vi "Diagnostics.Cleanup.vi"(8 "error in (no error)":errorcluster, 11 "State Variables":T1={"Comm"=refnum, "Parameters"={"Properties"={"Name"="", "CAN"={"CAN Interface"=enum."CAN1", "Baud Rate"=0, "Diagnostic Protocol"=enum."GMLAN", "Transport Protocol"=enum."ISO TP - Normal Mode", "Transmit ID"=0, "Receive ID"=0, "Transmit Extension"=2, "Receive Extension"=1, "Receive UUDT ID"=0, "Enable Stream"=TRUE, "VW TP Channel ID"=0, "Security"={"Source DLL Path"=path "", "Security Level"=0, "Target DLL Path"=path ""}, "Fill Frame"=FALSE, "Fill Byte"=255, "Termination"=FALSE}, "986x"={"Enable"=FALSE, "RIO Device"=0, "Bitfile"=path ""}, "Reads"=[], "Frames Lookup"=variant(enum16{"GMLAN", "KWP-2000", "UDS"} enum."GMLAN"), "Writes"=[], "DPIDs"=[], "DPID Lookup"=variant(u32 0), "DTC descriptor"={"DTC Byte Length"=2, "Status Byte Length"=1, "Add Data Byte Length"=1, "Byte Order"=enum."Motorola"}, "Created DTCs"=0}}, "ADCS Connection"={"Diag CAN Handle"=0, "Transport Protocol"=enum."ISO TP - Normal Mode", "Receive Address Extension"=0, "Transmit Address Extension"=0, "Receive CAN Id"=0, "Transmit CAN Id"=0, "Diag CAN Queue"=refnum, "Log Frames ?"=FALSE, "My TP Address"=0, "Other TP Address"=0, "T1"=0, "T2"=0, "T3"=0, "T4"=0, "Tx SN"=0, "Block Size"=0, "Rx SN"=0, "VW TP Initialized?"=FALSE, "Tx block no"=0, "baud rate"=0, "Interface"="", "Channel Diag CAN Handle"=0, "UDP Connection ID"=refnum, "TCP Connection ID"=refnum, "Target IP Addr"=0, "Source Address"=0, "Target Address"=0, "Send Header NACK?"=FALSE, "DLL Handle"=0, "NAD"=0, "Time Stamp read first"=0.0, "Time Stamp read last"=0.0, "Time Stamp write first"=0.0, "Time Stamp write last"=0.0, "Time Stamp write"=0.0, "Time Stamp read"=0.0}, "XNET References"={"Database"="", "GMLAN DPID Session"="", "Cluster"=""}, "XNETEngine (GMLAN)"=refnum, "Process"=refnum, "Reads"=refnum, "Writes"=refnum, "Cmds"=refnum, "DTCs"=refnum, "DTC Count"=refnum, "Status"=refnum, "Triggers"=refnum} {"Parameters"."Properties"."Writes"."Signals"."Byte Order" items=["Little Endian", "Big Endian"]; "Parameters"."Properties"."Writes"."Signals"."Data Type" items=["Signed", "Unsigned", "IEEE Float"]; "Parameters"."Properties"."CAN"."Fill Byte" format="%.0x"; "Parameters"."Properties"."CAN"."VW TP Channel ID" format="%.0x"; "Parameters"."Properties"."CAN"."Receive UUDT ID" format="%.0x"; "Parameters"."Properties"."CAN"."Receive Extension" format="%.0x"; "Parameters"."Properties"."CAN"."Transmit Extension" format="%.0x"; "Parameters"."Properties"."CAN"."Receive ID" format="%.0x"; "Parameters"."Properties"."CAN"."Transmit ID" format="%.0x"; "Parameters"."Properties"."Reads"."Signals"."Byte Order" items=["Little Endian", "Big Endian"]; "Parameters"."Properties"."Reads"."Signals"."Data Type" items=["Signed", "Unsigned", "IEEE Float"]}) -> (0 "error out":errorcluster)   [LabVIEW 2015, in "Diagnostics Addon Engine.lvlib"]
uses:
  Diagnostics Addon Engine.lvlib
  Types/Diagnostics.State.ctl
  <vilib>/NI/NIVS Inline Async API/_VS Inline Async API/Process/Process.lvclass
  <vilib>/NI/NIVS Addon Network Comm/Engine/VeriStand Comm.lvclass
  Shared/Types/SysDef.Compile.ctl
  Shared/Types/SysDef.Compile.Properties.ctl
  Shared/Types/CAN.ctl
  Shared/Types/CAN.Interface.ctl
  Shared/Types/Protocol.ctl
  Shared/Types/Transport.ctl
  Shared/Types/Security.ctl
  Shared/Types/986x.ctl
  Shared/Types/Frame.Compile.ctl
  Shared/Types/Type.ctl
  Shared/Types/Signal.ctl
  Shared/Types/DPID.ctl
  Shared/Types/DPID.Rate.ctl
  Shared/Types/DTCDescriptor.ctl
  <vilib>/Automotive Diagnostic Command Set/Diagnostic Transport.llb/Diag Reference.ctl
  <vilib>/Automotive Diagnostic Command Set/Diagnostic Transport.llb/Transport Protocol Selector.ctl
  <vilib>/Automotive Diagnostic Command Set/Diagnostic Transport.llb/Diag CAN Frame Log.ctl
  Types/XNET.Refs.ctl
  <vilib>/NI/AMC/Message Queue.ctl
  <vilib>/NI/AMC/Message.ctl
  <vilib>/NI/Tools/Keyed Array/KeyedArray.ctl
  <vilib>/NI/NIVS Inline Async API/_Data Access Engine/Access Type Classes/Write/Write.lvclass
  <vilib>/NI/NIVS Inline Async API/_Data Access Engine/Access Type Classes/Read/Read.lvclass
  <vilib>/NI/NIVS Inline Async API/_Data Access Engine/Access Type Classes/ReadWrite/ReadWrite.lvclass
  <vilib>/xnet/xnet.llb/XNET Database Close (Database).vi
  <vilib>/xnet/xnet.llb/XNET Database Delete (Cluster).vi
  Shared/SubVIs/Constants.vi
  <vilib>/addons/Automotive Diagnostic Command Set/NI_Automotive Diagnostic Command Set.lvlib
  <vilib>/NI/AMC/AMC.lvlib
  Shared/Diagnostics Addon Shared.lvlib
  <vilib>/NI/Tools/Keyed Array/Tools_KeyedArray.lvlib
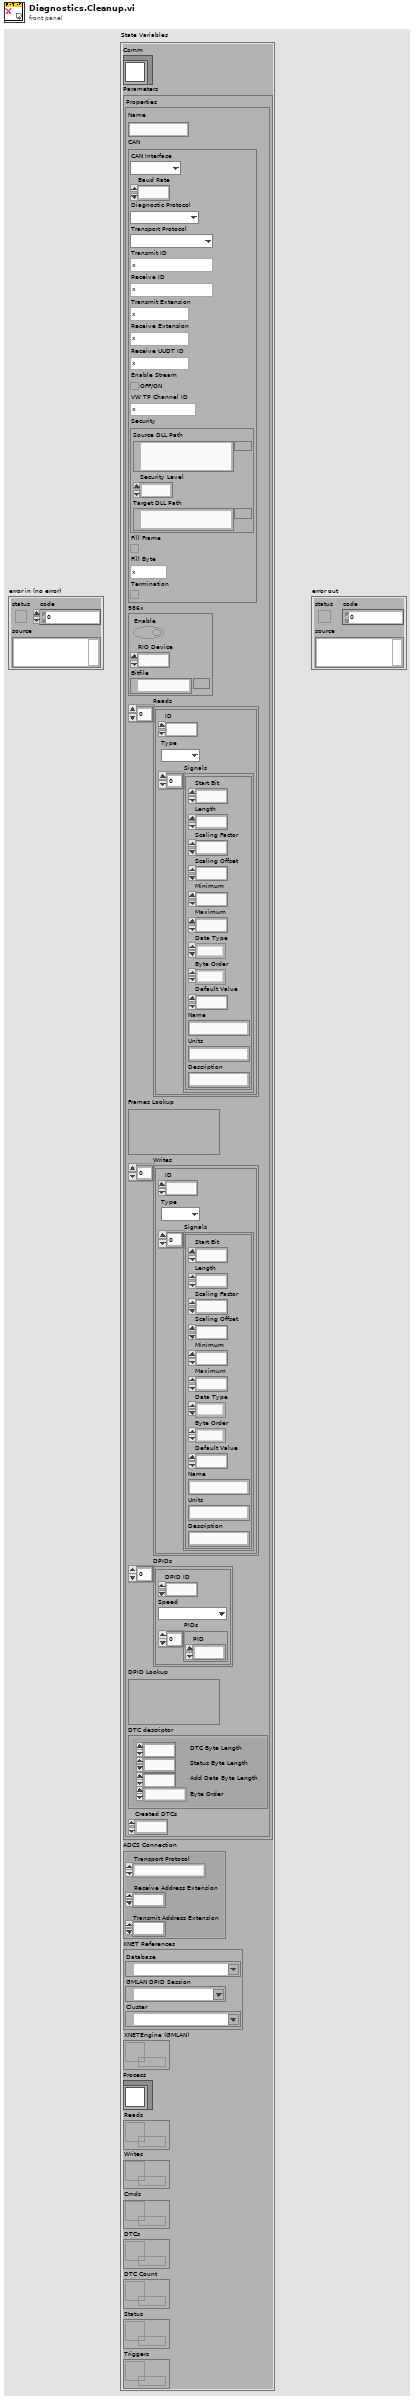
[diagram p1: front panel]
types:
  T1 = typedef "Diagnostics Addon Engine.lvlib/Diagnostics.State.ctl" = cluster{"Comm":refnum<class "VeriStand Comm.lvclass">, "Parameters":T2, "ADCS Connection":T16, "XNET References":T18, "XNETEngine (GMLAN)":T19, "Process":refnum<class "Process.lvclass">, "Reads":refnum<data-value>, "Writes":refnum<data-value>, "Cmds":refnum<data-value>, "DTCs":refnum<data-value>, "DTC Count":refnum<data-value>, "Status":refnum<data-value>, "Triggers":refnum<data-value>}
  T2 = typedef "Diagnostics Addon Shared.lvlib/SysDef.Compile.ctl" = cluster{"Properties":T3}
  T3 = typedef "Diagnostics Addon Shared.lvlib/SysDef.Compile.Properties.ctl" = cluster{"Name":string, "CAN":T4, "986x":T9, "Reads":T10[], "Frames Lookup":variant, "Writes":T10[], "DPIDs":T13[], "DPID Lookup":variant, "DTC descriptor":T15, "Created DTCs":u32}
  T4 = typedef "Diagnostics Addon Shared.lvlib/CAN.ctl" = cluster{"CAN Interface":T5, "Baud Rate":u32, "Diagnostic Protocol":T6, "Transport Protocol":T7, "Transmit ID":u32, "Receive ID":u32, "Transmit Extension":u8, "Receive Extension":u8, "Receive UUDT ID":u32, "Enable Stream":bool, "VW TP Channel ID":u32, "Security":T8, "Fill Frame":bool, "Fill Byte":u8, "Termination":bool}
  T5 = typedef "Diagnostics Addon Shared.lvlib/CAN.Interface.ctl" = enum16{"CAN0", "CAN1", "CAN2", "CAN3", "CAN4", "CAN5", "CAN6", "CAN7", "CAN8", "CAN9", "CAN10", "CAN11", "CAN12", "CAN13", "CAN14", "CAN15", "CAN16", "CAN17", "CAN18", "CAN19", "CAN20", "CAN21", "CAN22", "CAN23", "CAN24", "CAN25", "CAN26", "CAN27", "CAN28", "CAN29", "CAN30", "CAN31", "CAN32", "CAN33", "CAN34", "CAN35", "CAN36", "CAN37", "CAN38", "CAN39", "CAN40", "CAN41", "CAN42", "CAN43", "CAN44", "CAN45", "CAN46", "CAN47", "CAN48", "CAN49", "CAN50", "CAN51", "CAN52", "CAN53", "CAN54", "CAN55", "CAN56", "CAN57", "CAN58", "CAN59", "CAN60", "CAN61", "CAN62", "CAN63", "CAN 256 (Virtual)", "CAN 257 (Virtual)"}
  T6 = typedef "Diagnostics Addon Shared.lvlib/Protocol.ctl" = enum16{"GMLAN", "KWP-2000", "UDS", "User-Defined"}
  T7 = typedef "Diagnostics Addon Shared.lvlib/Transport.ctl" = enum16{"ISO TP - Normal Mode", "ISO TP - Mixed Mode", "VW TP 2.0", "Diagnostics on IP"}
  T8 = typedef "Diagnostics Addon Shared.lvlib/Security.ctl" = cluster{"Source DLL Path":path, "Security Level":u8, "Target DLL Path":path}
  T9 = typedef "Diagnostics Addon Shared.lvlib/986x.ctl" = cluster{"Enable":bool, "RIO Device":u16, "Bitfile":path}
  T10 = typedef "Diagnostics Addon Shared.lvlib/Frame.Compile.ctl" = cluster{"ID":u32, "Type":T11, "Signals":T12[]}
  T11 = typedef "Diagnostics Addon Shared.lvlib/Type.ctl" = enum16{"DID", "CDID", "PID", "CPID", "Read Memory", "Write Memory", "DTC Control", "IO Cmd", "IO Resp", "Routine Start Cmd", "Routine Start Resp", "Routine Request Cmd", "Routine Request Resp", "Routine Stop Cmd", "Routine Stop Resp", "UserDefined Cmd", "UserDefined Rsp"}
  T12 = typedef "Diagnostics Addon Shared.lvlib/Signal.ctl" = cluster{"Start Bit":u32, "Length":u32, "Scaling Factor":dbl, "Scaling Offset":dbl, "Minimum":dbl, "Maximum":dbl, "Data Type":u32, "Byte Order":u32, "Default Value":dbl, "Name":string, "Units":string, "Description":string}
  T13 = typedef "Diagnostics Addon Shared.lvlib/DPID.ctl" = cluster{"DPID ID":u8, "Speed":T14, "PIDs":u16[]}
  T14 = typedef "Diagnostics Addon Shared.lvlib/DPID.Rate.ctl" = enum16{"Slow", "Medium", "Fast"}
  T15 = typedef "Diagnostics Addon Shared.lvlib/DTCDescriptor.ctl" = cluster{"DTC Byte Length":i32, "Status Byte Length":i32, "Add Data Byte Length":i32, "Byte Order":enum16{"Motorola", "Intel"}}
  T16 = typedef "NI_Automotive Diagnostic Command Set.lvlib/Diag Reference.ctl" = cluster{"Diag CAN Handle":u32, "Transport Protocol":T17, "Receive Address Extension":u8, "Transmit Address Extension":u8, "Receive CAN Id":u32, "Transmit CAN Id":u32, "Diag CAN Queue":refnum<queue>, "Log Frames ?":bool, "My TP Address":u8, "Other TP Address":u8, "T1":u16, "T2":u16, "T3":u16, "T4":u16, "Tx SN":u8, "Block Size":u8, "Rx SN":u8, "VW TP Initialized?":bool, "Tx block no":u8, "baud rate":u32, "Interface":string, "Channel Diag CAN Handle":u32, "UDP Connection ID":refnum<k16>, "TCP Connection ID":refnum<k5>, "Target IP Addr":u32, "Source Address":u16, "Target Address":u16, "Send Header NACK?":bool, "DLL Handle":u32, "NAD":u8, "Time Stamp read first":dbl, "Time Stamp read last":dbl, "Time Stamp write first":dbl, "Time Stamp write last":dbl, "Time Stamp write":dbl, "Time Stamp read":dbl}
  T17 = typedef "NI_Automotive Diagnostic Command Set.lvlib/Transport Protocol Selector.ctl" = enum16{"ISO TP - Normal Mode", "ISO TP - Mixed Mode", "VW TP 2.0", "Diagnostics on IP", "ISO TP LIN"}
  T18 = typedef "Diagnostics Addon Engine.lvlib/XNET.Refs.ctl" = cluster{"Database":refnum<k21>, "GMLAN DPID Session":refnum<k21>, "Cluster":refnum<k21>}
  T19 = typedef "AMC.lvlib/Message Queue.ctl" = refnum<queue>
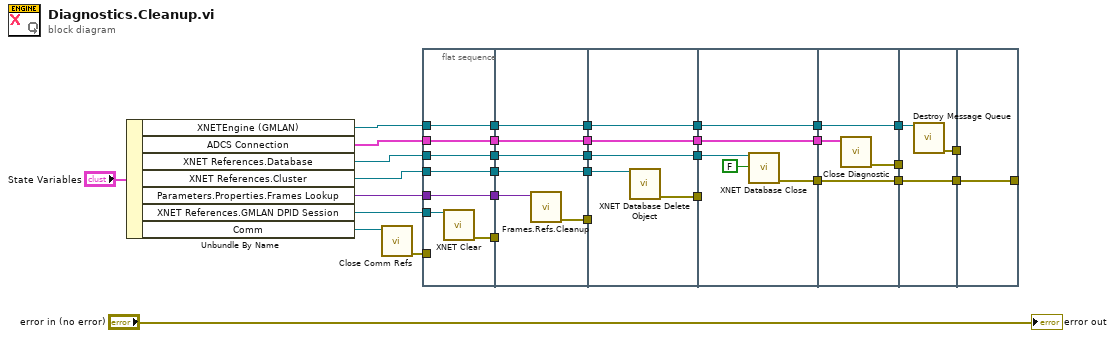
[diagram p0: block diagram]
diagram:
  n1 = Unbundle By Name("State Variables") -> ("XNETEngine (GMLAN)"=w23:T19, "ADCS Connection"=w17:T16, "XNET References.Database"=w8:refnum<k21>, "XNET References.Cluster"=w30:refnum<k21>, "Parameters.Properties.Frames Lookup"=w31:variant, "XNET References.GMLAN DPID Session"=w27:refnum<k21>, "Comm"=w1:refnum<class "VeriStand Comm.lvclass">)
  n2 = call <vilib>:"Close Comm Refs.vi"("Comm.lvclass"=w1) -> ("error out"=w22:errorcluster)  [unwired: 10 in]
  n3 = flat-sequence {
    tunnel: w30 -> [w39]
    tunnel: w31 -> [w40]
    tunnel: [w40] -> w29
    tunnel: [w39] -> w28
    tunnel: w27 -> [w38]
    tunnel: [w37] -> w26
    tunnel: [w36] -> w24
    tunnel: w23 -> [w36]
    tunnel: w22 -> [_]
    tunnel: [w35] -> w18
    tunnel: w17 -> [w35]
    tunnel: [w34] -> w9
    tunnel: w8 -> [w34]
    tunnel: [w46] -> w6
    tunnel: w29 -> [w44]
    tunnel: w28 -> [w46]
    tunnel: w26 -> [_]
    tunnel: [w45] -> w5
    tunnel: w24 -> [w45]
    tunnel: [w43] -> w4
    tunnel: w18 -> [w43]
    tunnel: [w42] -> w3
    tunnel: w9 -> [w42]
    tunnel: [w41] -> w2
    tunnel: w6 -> [w49]
    tunnel: [w51] -> w14
    tunnel: w5 -> [w51]
    tunnel: [w50] -> w12
    tunnel: w4 -> [w50]
    tunnel: [w48] -> w10
    tunnel: w3 -> [w48]
    tunnel: [w47] -> w7
    tunnel: w2 -> [_]
    tunnel: [w53] -> w15
    tunnel: w14 -> [w56]
    tunnel: [w56] -> w13
    tunnel: w12 -> [w55]
    tunnel: [w55] -> w11
    tunnel: w10 -> [w54]
    tunnel: w7 -> [_]
    tunnel: w15 -> [w60]
    tunnel: [w60] -> w20
    tunnel: w13 -> [w59]
    tunnel: [w59] -> w19
    tunnel: w11 -> [w58]
    tunnel: [w57] -> w16
    tunnel: w20 -> [w63]
    tunnel: [w63] -> w25
    tunnel: w19 -> [w62]
    tunnel: [w61] -> w21
    tunnel: w16 -> [_]
    tunnel: [w64] -> _
    tunnel: w25 -> [w64]
    tunnel: w21 -> [_]
    frame #0 {
      n4 = call <vilib>:"XNET Clear.vi"("session in"=w38) -> ("error out"=w37:errorcluster)  [unwired: 14 in]
    }
    frame #1 {
      n5 = call "Frames.Refs.Cleanup.vi"("Lookup"=w44) -> ("Array"=w41:errorcluster[])  [unwired: 10 in]
    }
    frame #2 {
      n6 = call-poly <vilib>:"XNET Database Delete Object.vi"("cluster in"=w49) -> ("error out"=w47:errorcluster)  [unwired: 14 in]
    }
    frame #3 {
      n7 = call-poly <vilib>:"XNET Database Close.vi"("database in"=w54, "close all? (true)"=FALSE) -> ("error out"=w53:errorcluster)  [unwired: 13 in]
    }
    frame #4 {
      n8 = call <vilib>:"Close Diagnostic.vi"("diag ref in"=w58) -> ("error out"=w57:errorcluster)  [unwired: 10 in]
    }
    frame #5 {
      n9 = call <vilib>:"Destroy Message Queue.vi"("message queue in"=w62) -> ("error out"=w61:errorcluster)  [unwired: 12 in, 2 out]
    }
    frame #6 {
    }
  }
  "error out" <- "error in (no error)"
